vi "Write to Grad PieChart.vi"(8 "error in (no error)":errorcluster caption="错误输入（无错误）", 10 "Grad PieChart":picture, 11 "Gradient PieChart输入":refnum<class "Gradient PieChart.lvclass">) -> (0 "error out":errorcluster caption="错误输出", 3 "Gradient PieChart输出":refnum<class "Gradient PieChart.lvclass">)   [LabVIEW 2012, in "Gradient PieChart.lvclass"]
uses:
  Gradient PieChart.lvclass
  Gradient PieChart.lvclass/Gradient PieChart.ctl
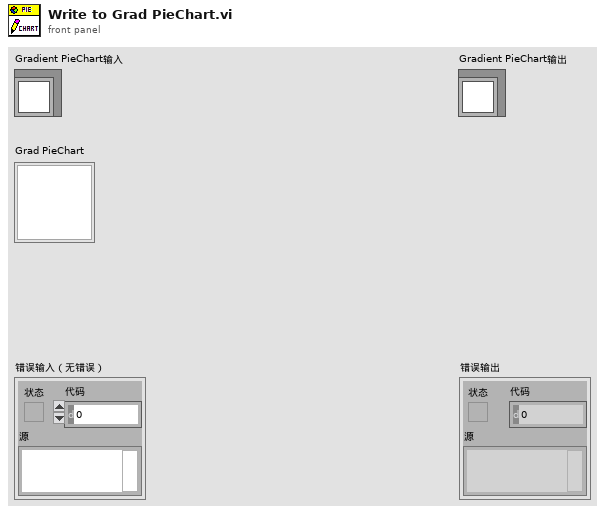
[diagram p1: front panel]
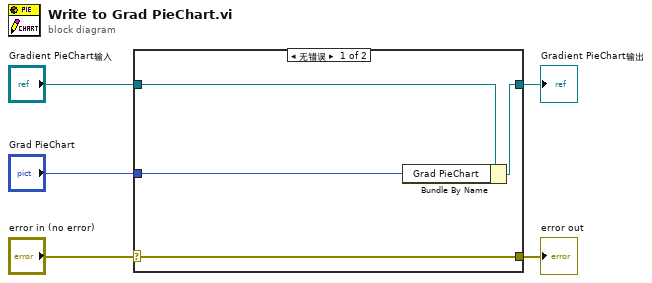
[diagram p0: block diagram]
diagram:
  n1 = case shown="无错误" "error in (no error)" {
    selector: "error in (no error)" -> [w9 w10]
    tunnel: [w9 w10] -> w4
    tunnel: [w7 w11] -> w2
    tunnel: "Gradient PieChart输入" -> [w8 w11]
    tunnel: "Grad PieChart" -> [w6 _]
    frame No Error {
      n2 = Bundle By Name(cluster=w8, "Grad PieChart"=w6) -> (w7:refnum<class "Gradient PieChart.lvclass">)
    }
    frame Error {
    }
  }
  "error out" <- w4
  "Gradient PieChart输出" <- w2
